vi "SMU Create Adv Seq.vi"(8 "error in (no error)":errorcluster, 10 "JSONCluster":T1, 11 "IVI Refnum in":refnum<k15>) -> (0 "error out":errorcluster, 3 "IVI Refnum out":refnum<k15>)   [LabVIEW 2019, in "SupportVIs.lvlib"]
uses:
  SupportVIs.lvlib
  JSONCluster.ctl
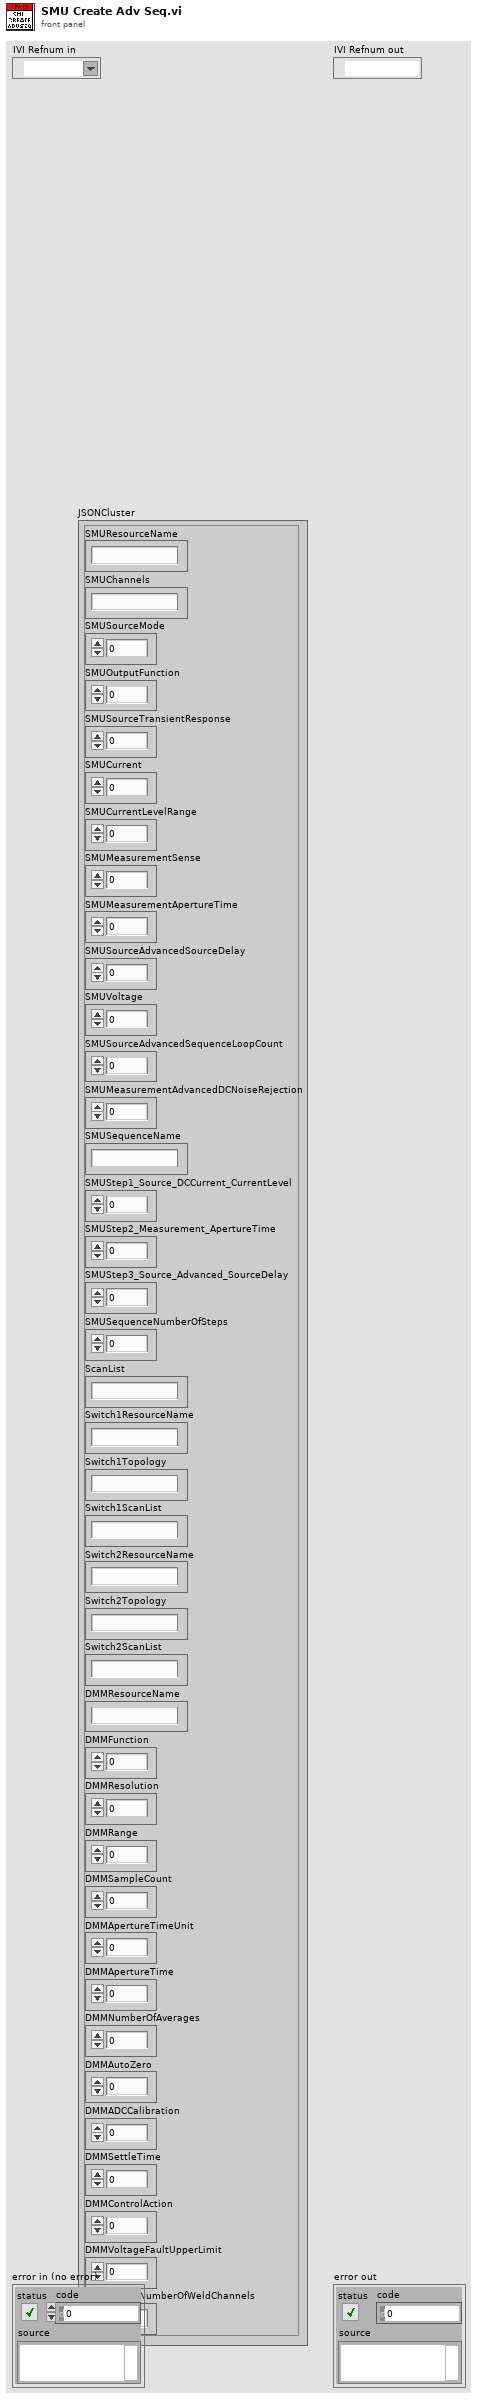
[diagram p1: front panel]
types:
  T1 = typedef "JSONCluster.ctl" = cluster{"SMUResourceName":string, "SMUChannels":string, "SMUSourceMode":i32, "SMUOutputFunction":i32, "SMUSourceTransientResponse":i32, "SMUCurrent":dbl, "SMUCurrentLevelRange":dbl, "SMUMeasurementSense":i32, "SMUMeasurementApertureTime":dbl, "SMUSourceAdvancedSourceDelay":dbl, "SMUVoltage":dbl, "SMUSourceAdvancedSequenceLoopCount":i32, "SMUMeasurementAdvancedDCNoiseRejection":i32, "SMUSequenceName":string, "SMUStep1_Source_DCCurrent_CurrentLevel":i32, "SMUStep2_Measurement_ApertureTime":i32, "SMUStep3_Source_Advanced_SourceDelay":i32, "SMUSequenceNumberOfSteps":i32, "ScanList":string, "Switch1ResourceName":string, "Switch1Topology":string, "Switch1ScanList":string, "Switch2ResourceName":string, "Switch2Topology":string, "Switch2ScanList":string, "DMMResourceName":string, "DMMFunction":i32, "DMMResolution":dbl, "DMMRange":dbl, "DMMSampleCount":i32, "DMMApertureTimeUnit":i32, "DMMApertureTime":dbl, "DMMNumberOfAverages":i32, "DMMAutoZero":i32, "DMMADCCalibration":i32, "DMMSettleTime":dbl, "DMMControlAction":i32, "DMMVoltageFaultUpperLimit":dbl, "ApplicationNumberOfWeldChannels":i32}
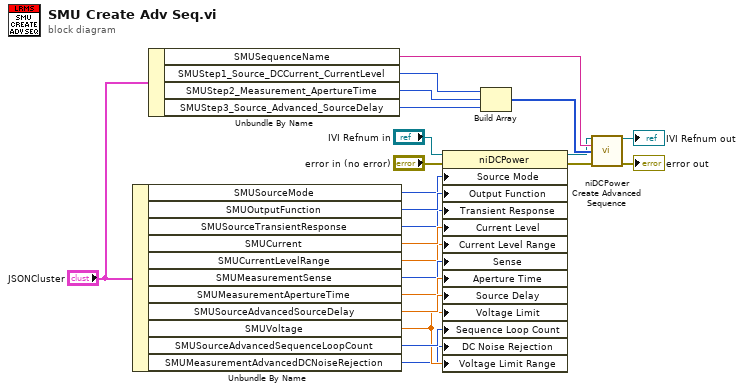
[diagram p0: block diagram]
diagram:
  n1 = Unbundle By Name("JSONCluster") -> ("SMUSourceMode"=w10:i32, "SMUOutputFunction"=w11:i32, "SMUSourceTransientResponse"=w7:i32, "SMUCurrent"=w19:dbl, "SMUCurrentLevelRange"=w8:dbl, "SMUMeasurementSense"=w9:i32, "SMUMeasurementApertureTime"=w20:dbl, "SMUSourceAdvancedSourceDelay"=w21:dbl, "SMUVoltage"=w13:dbl, "SMUSourceAdvancedSequenceLoopCount"=w18:i32, "SMUMeasurementAdvancedDCNoiseRejection"=w12:i32)
  n2 = Unbundle By Name("JSONCluster") -> ("SMUSequenceName"=w23:string, "SMUStep1_Source_DCCurrent_CurrentLevel"=w15:i32, "SMUStep2_Measurement_ApertureTime"=w16:i32, "SMUStep3_Source_Advanced_SourceDelay"=w17:i32)
  n3 = property class="niDCPower"(reference="IVI Refnum in", error in="error in (no error)", "Source Mode"=w10, "Output Function"=w11, "Transient Response"=w7, "Current Level"=w19, "Current Level Range"=w8, "Sense"=w9, "Aperture Time"=w20, "Source Delay"=w21, "Voltage Limit"=w13, "Sequence Loop Count"=w18, "DC Noise Rejection"=w12, "Voltage Limit Range"=w13) -> (reference out=w3:refnum<k15>, error out=w4:errorcluster)
  n4 = Build Array(w15, w16, w17) -> (w14:i32[])
  n5 = call <instrlib>:"niDCPower Create Advanced Sequence.vi"("instrument handle"=w3, "sequence name"=w23, "advanced sequence properties"=w14, "error in (no error)"=w4) -> ("instrument handle out"=→"IVI Refnum out":refnum<k15>, "error out"=→"error out":errorcluster)  [unwired: 10 in]
